vi "Eliminate V offsets with OCO.vi"() -> ()   [LabVIEW 2013]
doc: "Offset Compensated Ohms improves the accuracy of resistance measurements by removing voltage offsets from the measurement. Offset Compensated Ohms is useful for resistance measurements under 10K Ohms.\nThis example acquires a 2-wire or 4-wire resistance measurement. After specifying the instrument descriptor, select the function, range, and resolution. Turning on Offset Compensated Ohms will perform an offset compensation adjustment on the resistance measurement."
uses:
  <instrlib>/niDMM/nidmm.llb/niDMM Function.ctl
  <instrlib>/niDMM/nidmm.llb/niDMM Offset Comp Ohms.ctl
  <instrlib>/niDMM/nidmm.llb/niDMM Powerline Frequency.ctl
  <instrlib>/niDMM/nidmm.llb/niDMM Resolution in Digits.ctl
  <instrlib>/niDMM/nidmm.llb/niDMM Configure Measurement Digits.vi
panel:
  in  "Resolution in Digits":T1=5.5 items=["3 1/2"=3.5, "4 1/2"=4.5, "5 1/2"=5.5, "6 1/2"=6.5, "7 1/2"=7.5]
  in  "Powerline Frequency":T2
  in  "Offset Compensated Ohms":T3=1 items=["Off", "On"]
  in  "Measurement Type":T4=enum."4-wire Resistance"
  out "Signal Out of Range":bool
  in  "Device Name":refnum<k15>="Dev1"
  in  "Range":dbl=1000.0 format="%.2p"
  out "Measurement (Ohms)":dbl format="%_7p"
  # "For instructions select File >> VI Properties >> Documentation"
  # "Configuration"
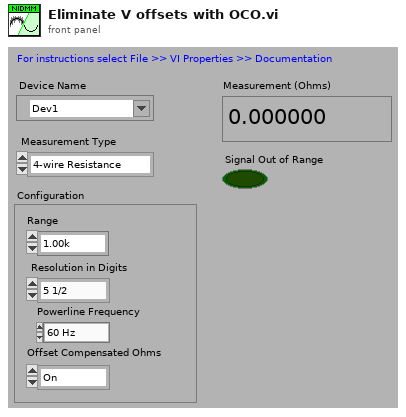
[diagram p1: front panel]
types:
  T1 = typedef "niDMM Resolution in Digits.ctl" = dbl
  T2 = typedef "niDMM Powerline Frequency.ctl" = enum16{"60 Hz", "50 Hz"}
  T3 = typedef "niDMM Offset Comp Ohms.ctl" = i32
  T4 = typedef "niDMM Function.ctl" = enum16{"DC Volts", "AC Volts", "DC Current", "AC Current", "2-wire Resistance", "4-wire Resistance", "Diode", "Frequency", "Period", "AC Volts DC Coupled", "Capacitance", "Inductance", "Temperature"}
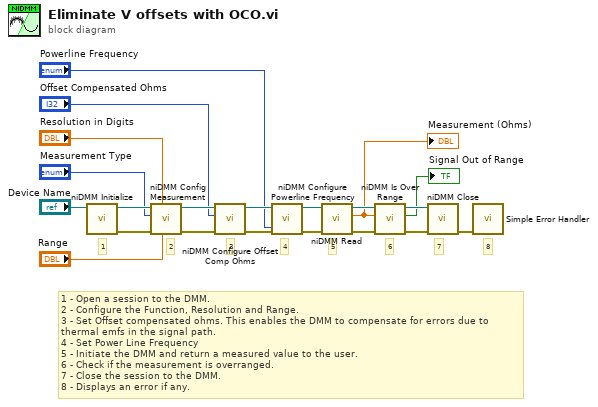
[diagram p0: block diagram]
diagram:
  # "8"
  # "7"
  # "3"
  # "1 - Open a session to the DMM.\n2 - Configure the Function, Resolution and Range.\n3 - Set Offset compensated ohms. This enables the DMM to compensate for errors due to thermal emfs in the signal path.\n4 - Set Power Line Frequency\n5 - Initiate the DMM and return a measured value to the user.\n6 - Check if the measurement is overranged.\n7 - Close the session to the DMM.\n8 - Displays an error if any."
  # "1"
  # "6"
  # "5"
  # "4"
  # "2"
  n1 = call <instrlib>:"niDMM Initialize.vi"("Instrument Descriptor"="Device Name") -> ("error out"=w20:errorcluster, "instrument handle out"=w21:refnum<k15>)  [unwired: 9 in]
  n2 = call-poly <instrlib>:"niDMM Config Measurement.vi"("Range"="Range", "Resolution in Digits"="Resolution in Digits", "error in (no error)"=w20, "Function"="Measurement Type", "instrument handle"=w21) -> ("error out"=w16:errorcluster, "instrument handle out"=w15:refnum<k15>)  [unwired: 5 in]
  n3 = call <instrlib>:"niDMM Configure Offset Comp Ohms.vi"("error in (no error)"=w16, "Offset Compensated Ohms"="Offset Compensated Ohms", "instrument handle"=w15) -> ("error out"=w6:errorcluster, "instrument handle out"=w5:refnum<k15>)  [unwired: 7 in]
  n4 = call <instrlib>:"niDMM Configure Powerline Frequency.vi"("Powerline Frequency"="Powerline Frequency", "error in (no error)"=w6, "instrument handle"=w5) -> ("error out"=w7:errorcluster, "instrument handle out"=w4:refnum<k15>)  [unwired: 7 in]
  n5 = call <instrlib>:"niDMM Read.vi"("error in (no error)"=w7, "instrument handle"=w4) -> ("error out"=w13:errorcluster, "Measurement"=w10:dbl, "instrument handle out"=w14:refnum<k15>)  [unwired: 7 in]
  "Measurement (Ohms)" <- w10
  n6 = call <instrlib>:"niDMM Is Over Range.vi"("error in (no error)"=w13, "Measurement"=w10, "instrument handle"=w14) -> ("error out"=w11:errorcluster, "Over Range?"=→"Signal Out of Range":bool, "instrument handle out"=w12:refnum<k15>)  [unwired: 6 in]
  n7 = call <instrlib>:"niDMM Close.vi"("error in (no error)"=w11, "instrument handle"=w12) -> ("error out"=w8:errorcluster)  [unwired: 9 in]
  n8 = call <vilib>:"Simple Error Handler.vi"("error in (no error)"=w8) -> ()  [unwired: 4 in, 5 out]
